vi "未命名 2.vi"() -> ()   [LabVIEW 2020]
panel:
  out "添加的数组":cluster{dbl[], dbl[]}[](array[cluster])
  in  "停止":bool
  in  "文件（使用对话框）":path
  out "XY graph 2":cluster{"Wavenumber":dbl[], "Data":dbl[]}[](graph)
  out "XY graph":cluster{"Wavenumber":dbl[], "Data":dbl[]}[](graph)
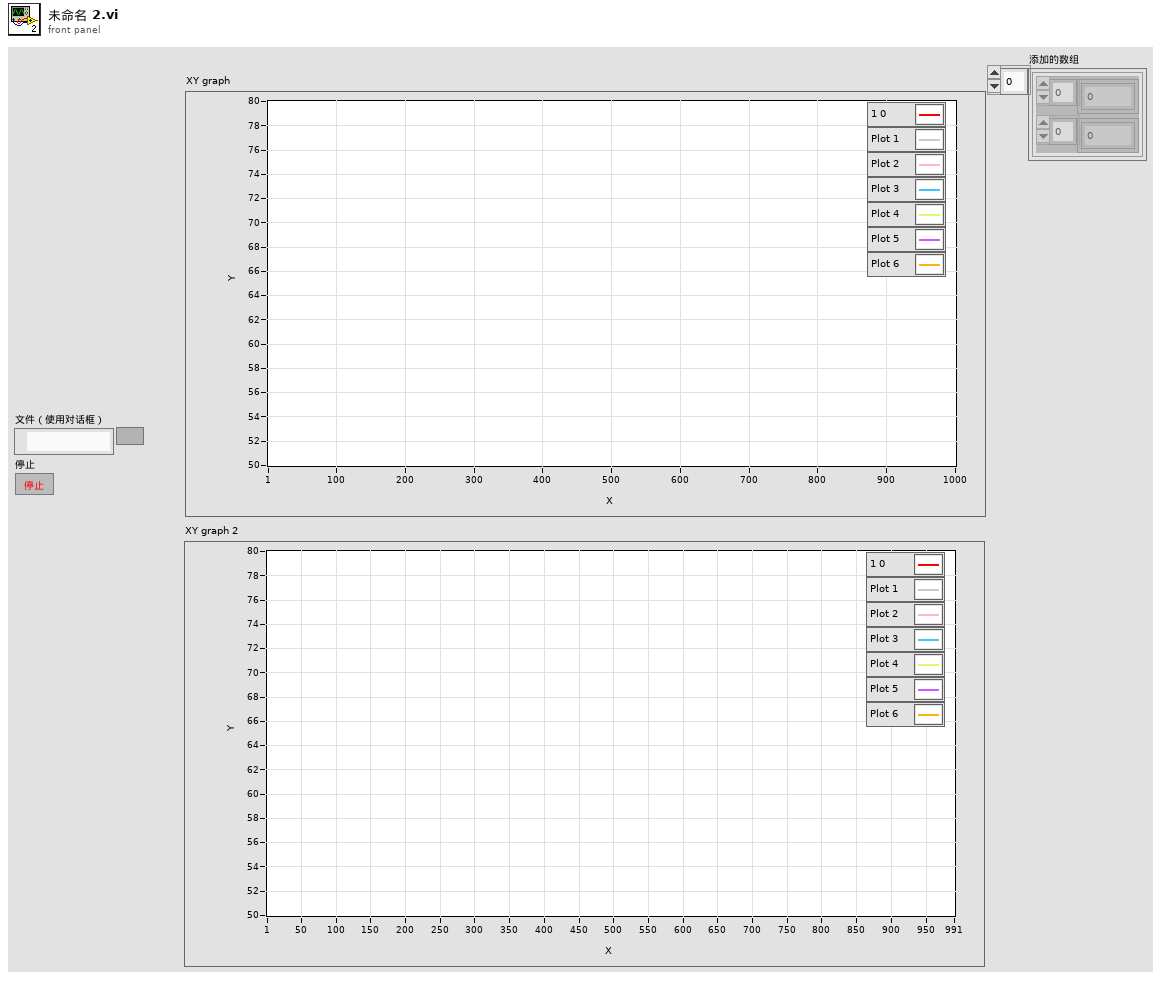
[diagram p1: front panel]
types:
  T1 = enum16{"big-endian, network order", "native, host order", "little-endian"}
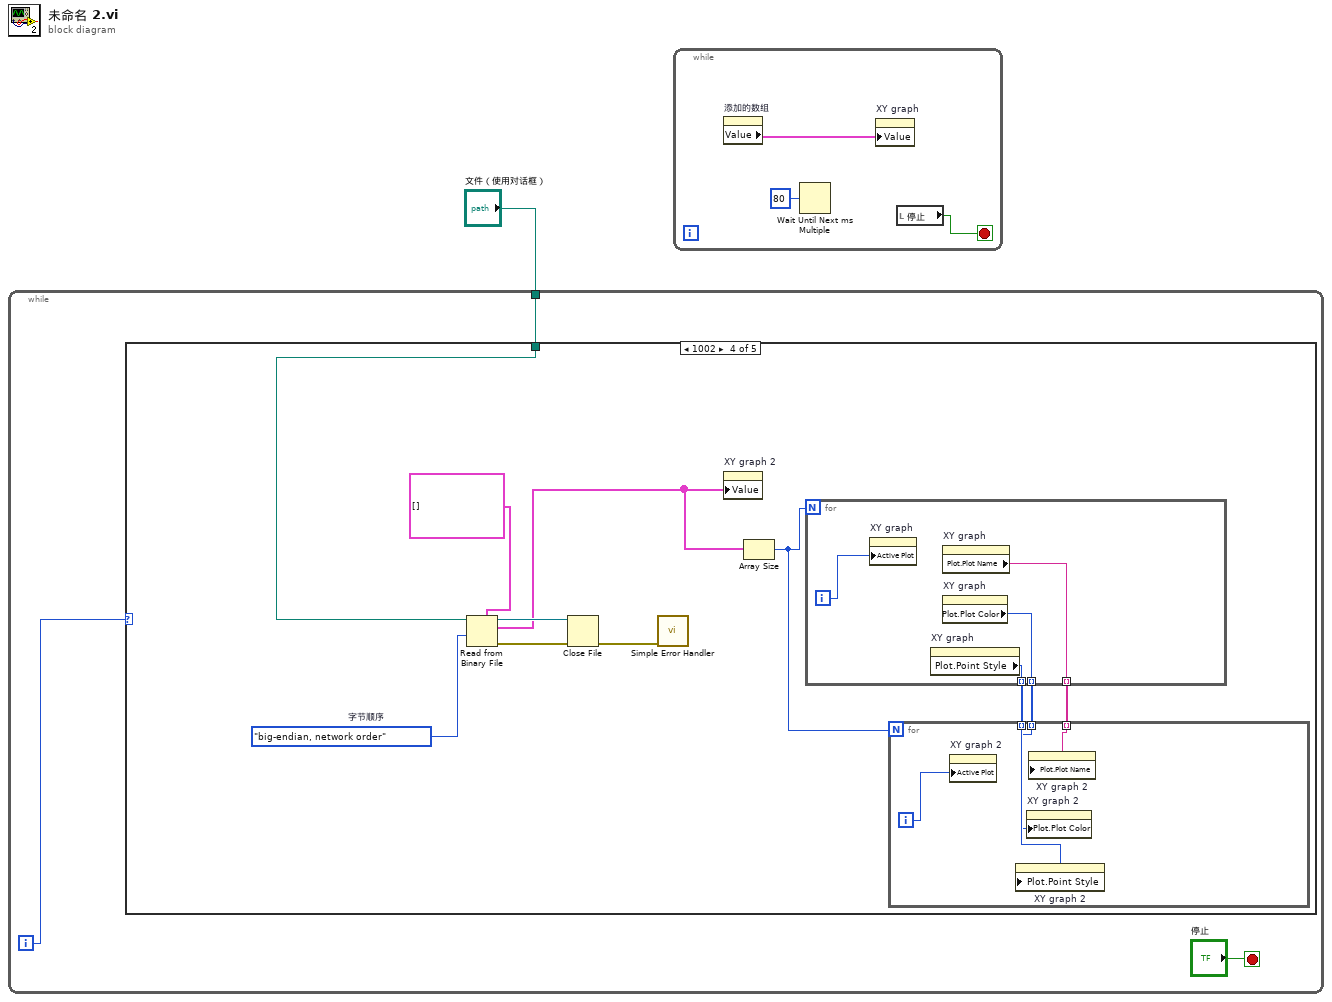
[diagram p0: block diagram]
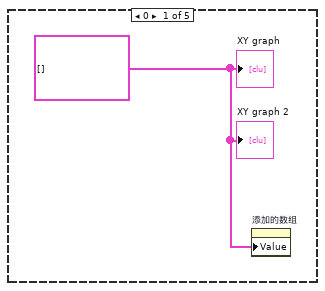
[diagram p2: hidden frame]
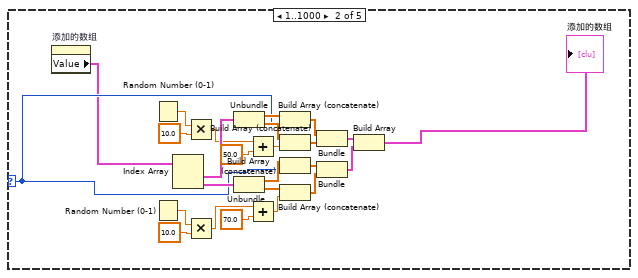
[diagram p3: hidden frame]
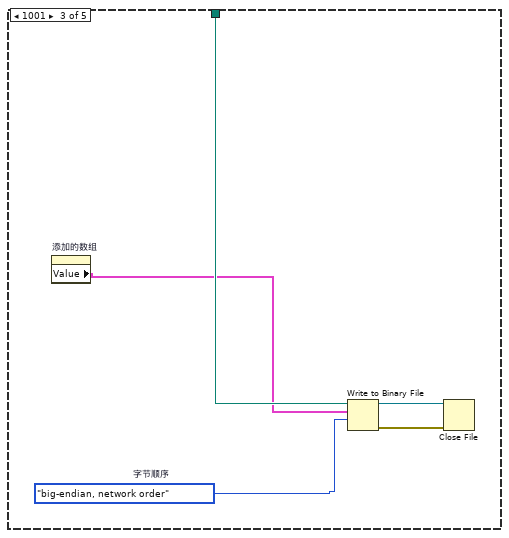
[diagram p4: hidden frame]
diagram:
  n1 = while {
    tunnel: "文件（使用对话框）" -> [w3]
    i -> [w4]
    stop <- "停止" stop-if-true
    n2 = case shown="1002" w4 {
      selector: w4 -> [_ w17 _ _ _]
      tunnel: w3 -> [_ _ w32 w41 _]
      frame 0 {
        w5 = cluster{dbl[], dbl[]}[] []
        n3 = property on="添加的数组" class="Arr (严格)"("Value"=w5) -> ()  [unwired: 2 in, 2 out]
        "XY graph" <- w5
        "XY graph 2" <- w5
      }
      frame 1..1000 {
        n4 = property on="添加的数组" class="Arr (严格)"() -> ("Value"=w6:cluster{dbl[], dbl[]}[])  [unwired: 2 in, 2 out]
        n5 = Random Number (0-1)() -> (number: 0 to 1=w16:dbl)
        n6 = Random Number (0-1)() -> (number: 0 to 1=w11:dbl)
        n7 = Index Array(array=w6) -> (element #1=w30:cluster{dbl[], dbl[]}, element #2=w25:cluster{dbl[], dbl[]})  [unwired: 2 in]
        n8 = Multiply(x=w16, y=10.0) -> (x*y=w14:dbl)
        n9 = Multiply(x=w11, y=10.0) -> (x*y=w10:dbl)
        n10 = Unbundle(w30) -> (w29:dbl[], w28:dbl[])
        n11 = Unbundle(w25) -> (w26:dbl[], w27:dbl[])
        n12 = Add(x=w14, y=50.0) -> (x+y=w8:dbl)
        n13 = Add(x=w10, y=70.0) -> (x+y=w7:dbl)
        n14 = Build Array (concatenate)(w29, w17) -> (w24:dbl[])
        n15 = Build Array (concatenate)(w28, w8) -> (w23:dbl[])
        n16 = Build Array (concatenate)(w26, w17) -> (w22:dbl[])
        n17 = Build Array (concatenate)(w27, w7) -> (w21:dbl[])
        n18 = Bundle(w24, w23) -> (w20:cluster{dbl[], dbl[]})  [unwired: 1 in]
        n19 = Bundle(w22, w21) -> (w19:cluster{dbl[], dbl[]})  [unwired: 1 in]
        n20 = Build Array(w20, w19) -> (→"添加的数组":cluster{dbl[], dbl[]}[])
      }
      frame 1001 {
        w33 = T1."big-endian, network order"  # 字节顺序
        n21 = property on="添加的数组" class="Arr (严格)"() -> ("Value"=w31:cluster{dbl[], dbl[]}[])  [unwired: 2 in, 2 out]
        n22 = Write to Binary File(file (use dialog)=w32, data=w31, 9:w33) -> (refnum out=w35:refnum<file>, error out=w34:errorcluster)  [unwired: 3 in, 1 out]
        n23 = Close File(refnum=w35, error in=w34) -> ()  [unwired: 2 out]
      }
      frame 1002 {
        w44 = T1."big-endian, network order"  # 字节顺序
        n24 = Read from Binary File(5:cluster{dbl[], dbl[]}[] [], 9:w44, 11:w41) -> (0:w45:errorcluster, 2:w36:cluster{dbl[], dbl[]}[], 3:w46:refnum<file>)  [unwired: 3 in, 1 out]
        n25 = Close File(refnum=w46, error in=w45) -> (error out=w43:errorcluster)  [unwired: 1 out]
        n26 = call <vilib>:"Simple Error Handler.vi"("error in (no error)"=w43) -> ()  [unwired: 4 in, 5 out]
        n27 = property on="XY graph 2" class="XYGraph (严格)"("Value"=w36) -> ()  [unwired: 2 in, 2 out]
        n28 = Array Size(array=w36) -> (size(s)=w40:i32)
        n29 = for {
          N: w40 -> [_]
          tunnel: [w53] -> w39 mode=indexing
          tunnel: [w52] -> w38 mode=indexing
          tunnel: [w51] -> w37 mode=indexing
          i -> [w54]
          n30 = property on="XY graph" class="XYGraph (严格)"("Active Plot"=w54) -> ()  [unwired: 2 in, 2 out]
          n31 = property on="XY graph" class="XYGraph (严格)"() -> ("Plot.Point Style"=w53:u8)  [unwired: 2 in, 2 out]
          n32 = property on="XY graph" class="XYGraph (严格)"() -> ("Plot.Plot Name"=w52:string)  [unwired: 2 in, 2 out]
          n33 = property on="XY graph" class="XYGraph (严格)"() -> ("Plot.Plot Color"=w51:u32)  [unwired: 2 in, 2 out]
        }
        n34 = for {
          N: w40 -> [_]
          tunnel: w39 -> [w49] mode=indexing
          tunnel: w38 -> [w48] mode=indexing
          tunnel: w37 -> [w47] mode=indexing
          i -> [w50]
          n35 = property on="XY graph 2" class="XYGraph (严格)"("Active Plot"=w50) -> ()  [unwired: 2 in, 2 out]
          n36 = property on="XY graph 2" class="XYGraph (严格)"("Plot.Point Style"=w49) -> ()  [unwired: 2 in, 2 out]
          n37 = property on="XY graph 2" class="XYGraph (严格)"("Plot.Plot Color"=w47) -> ()  [unwired: 2 in, 2 out]
          n38 = property on="XY graph 2" class="XYGraph (严格)"("Plot.Plot Name"=w48) -> ()  [unwired: 2 in, 2 out]
        }
      }
      frame 1003, Default {
      }
    }
  }
  n39 = while {
    stop <- w56 stop-if-true
    n40 = property on="添加的数组" class="Arr (严格)"() -> ("Value"=w57:cluster{dbl[], dbl[]}[])  [unwired: 2 in, 2 out]
    n41 = Wait Until Next ms Multiple(millisecond multiple=u32 80 ("毫秒倍数")) -> ()  [unwired: 1 out]
    n42 = property on="XY graph" class="XYGraph (严格)"("Value"=w57) -> ()  [unwired: 2 in, 2 out]
    n43 = local read "停止"() -> (w56:bool)
  }
